vi "Load_Digital_OP.vi"(7 "ReadOnlyIn":T11={"Qref"={"ValveCTR"=refnum, "Error"=refnum}, "UI_EN"=FALSE, "UserEventREF"={"TimeBasedProducer"={"Reg"=refnum, "Ref"=refnum}, "TimeBasedTempRead"={"Reg"=refnum, "Ref"=refnum}}, "UI_REF"=variant(cluster{} {}), "Paths"={"Log_Dir"=path "", "TempLog"=path "", "WateringLog"=path "", "Error"=path "", "Settings_Dir"=path "", "CFG.ini"=path "", "Plant_Digital_OP"=path "", "TimeTable"=path "", "Consol_Dir"=path "", "Input"=path "", "Output"=path "", "Timeout"=path "", "TimeoutTable"=path "", "Ch_Stat"=path "", "Temp"=path ""}, "PI_REF"={"IO"=enum."Remote", "Interface"=enum."Serial", "LINX Device Config"={"Interface"=enum."Serial", "COM Port"="COM13", "TCP Configuration"={"IP Address"="", "Port"=0}, "Device Family"=1, "Device ID"=1, "Device Name"="myRIO-1900", "TCP Ref"=refnum, "Channels"={"DI"=[0, 1, 2, 3, 4, 5, 6, 7, 8, 9, 10, 11, 12, 13, 14, 15, 16, 17, 18, 19, 20, 21, 22, 23, 24, 25, 26, 27, 28, 29, 30, 31, 32, 33, 34, 35, 36, 37, 38, 39, 40, 41, 42, 43, 44, 45, 46], "DO"=[0, 1, 2, 3, 4, 5, 6, 7, 8, 9, 10, 11, 12, 13, 14, 15, 16, 17, 18, 19, 20, 21, 22, 23, 24, 25, 26, 27, 28, 29, 30, 31, 32, 33, 34, 35, 36, 37, 38, 39, 40, 41, 42, 43, 44, 45, 46], "AI"=[0, 1, 2, 3, 4, 5, 6, 7, 8, 9, 10, 11], "AO"=[], "PWM"=[3, 5, 6, 9, 10], "QE"=[], "UART"=[0, 1], "I2C 2"=[0], "SPI"=[0], "CAN"=[], "Servo"=[], "AI Ref (V)"=0.0, "AI Resolution (Bits)"=0, "AO Ref (V)"=0.0, "AO Resolution (Bits)"=0}}}, "CFG"={"ProducerEn_PC"=FALSE, "Producer_PC_ms"=0, "ProducerEn_PI"=FALSE, "Producer_PI_ms"=0, "TempLogInterval"=15, "SystemResetTime"=0.0}} {"CFG"."SystemResetTime" format="%<%H:%M:%S>t"}, 8 "Error In":errorcluster, 9 "Oper":enum16{"FromFile", "FromMem"}(ring), 10 "Plants_Digital_OP":refnum<vi>, 11 "Read_WriteIN":T2={"Time Table"=[{"Set Time"=0.0, "Control"=enum."Time", "Duration[S]"=3.0, "Liter"=0.0, "Plant Name."="", "Watered"=FALSE, "Su"=FALSE, "Mo"=FALSE, "Tu"=FALSE, "We"=FALSE, "Th"=FALSE, "Fr"=FALSE, "Sa"=FALSE}, {"Set Time"=0.0, "Control"=enum."Time", "Duration[S]"=5.0, "Liter"=0.0, "Plant Name."="", "Watered"=FALSE, "Su"=FALSE, "Mo"=FALSE, "Tu"=FALSE, "We"=FALSE, "Th"=FALSE, "Fr"=FALSE, "Sa"=FALSE}, {"Set Time"=0.0, "Control"=enum."Time", "Duration[S]"=5.0, "Liter"=0.0, "Plant Name."="", "Watered"=FALSE, "Su"=FALSE, "Mo"=FALSE, "Tu"=FALSE, "We"=FALSE, "Th"=FALSE, "Fr"=FALSE, "Sa"=FALSE}], "Plants_Digital_OP"=[], "delta_ms_w_Index"={"delta_ms"=[], "Index"=[], "RunArray"=[]}, "TimeOutInfo"={"Timeout"=0, "ValveCTR"={"State"=enum."Open Valve", "Channel No"=0, "Duration[S]"=0.0}, "Index"=0}, "LoopName"=""} {"TimeOutInfo"."ValveCTR"."Channel No" items=["7"=7, "11"=11, "12"=12, "13"=13, "15"=15, "16"=16, "18"=18, "29"=29, "32"=32, "33"=33, "35"=35, "36"=36, "37"=37, "38"=38, "40"=40]; "delta_ms_w_Index"."RunArray"."Channel No" items=["7"=7, "11"=11, "12"=12, "13"=13, "15"=15, "16"=16, "18"=18, "29"=29, "32"=32, "33"=33, "35"=35, "36"=36, "37"=37, "38"=38, "40"=40]; "Plants_Digital_OP"."Channel No" items=["7"=7, "11"=11, "12"=12, "13"=13, "15"=15, "16"=16, "18"=18, "29"=29, "32"=32, "33"=33, "35"=35, "36"=36, "37"=37, "38"=38, "40"=40]; "Time Table"."Liter" min=0.0; "Time Table"."Set Time" format="%<%H:%M:%S>t"; "Time Table"."Duration[S]" min=0.0}) -> (0 "Error Out":errorcluster, 2 "ValidCh":T1[](array[typedef]) items=["7"=7, "11"=11, "12"=12, "13"=13, "15"=15, "16"=16, "18"=18, "29"=29, "32"=32, "33"=33, "35"=35, "36"=36, "37"=37, "38"=38, "40"=40], 3 "Read_WriteIOUT":T2={"Time Table"=[{"Set Time"=0.0, "Control"=enum."Time", "Duration[S]"=3.0, "Liter"=0.0, "Plant Name."="", "Watered"=FALSE, "Su"=FALSE, "Mo"=FALSE, "Tu"=FALSE, "We"=FALSE, "Th"=FALSE, "Fr"=FALSE, "Sa"=FALSE}, {"Set Time"=0.0, "Control"=enum."Time", "Duration[S]"=5.0, "Liter"=0.0, "Plant Name."="", "Watered"=FALSE, "Su"=FALSE, "Mo"=FALSE, "Tu"=FALSE, "We"=FALSE, "Th"=FALSE, "Fr"=FALSE, "Sa"=FALSE}, {"Set Time"=0.0, "Control"=enum."Time", "Duration[S]"=5.0, "Liter"=0.0, "Plant Name."="", "Watered"=FALSE, "Su"=FALSE, "Mo"=FALSE, "Tu"=FALSE, "We"=FALSE, "Th"=FALSE, "Fr"=FALSE, "Sa"=FALSE}], "Plants_Digital_OP"=[], "delta_ms_w_Index"={"delta_ms"=[], "Index"=[], "RunArray"=[]}, "TimeOutInfo"={"Timeout"=0, "ValveCTR"={"State"=enum."Open Valve", "Channel No"=0, "Duration[S]"=0.0}, "Index"=0}, "LoopName"=""} {"TimeOutInfo"."ValveCTR"."Channel No" items=["7"=7, "11"=11, "12"=12, "13"=13, "15"=15, "16"=16, "18"=18, "29"=29, "32"=32, "33"=33, "35"=35, "36"=36, "37"=37, "38"=38, "40"=40]; "delta_ms_w_Index"."RunArray"."Channel No" items=["7"=7, "11"=11, "12"=12, "13"=13, "15"=15, "16"=16, "18"=18, "29"=29, "32"=32, "33"=33, "35"=35, "36"=36, "37"=37, "38"=38, "40"=40]; "Plants_Digital_OP"."Channel No" items=["7"=7, "11"=11, "12"=12, "13"=13, "15"=15, "16"=16, "18"=18, "29"=29, "32"=32, "33"=33, "35"=35, "36"=36, "37"=37, "38"=38, "40"=40]; "Time Table"."Liter" min=0.0; "Time Table"."Set Time" format="%<%H:%M:%S>t"; "Time Table"."Duration[S]" min=0.0})   [LabVIEW 2014, in "TimeBasedProd.lvlib"]
uses:
  TimeBasedProd.lvlib
  TypeDef/Read_Write.ctl
  TimeTable/TypeDef/Time_Table.ctl
  TimeTable/TypeDef/Time_Table_CTR.ctl
  TypeDef/Plant_OP_Map.ctl
  TypeDef/Plant_OP_Map_CTR.ctl
  ValveCTRL/TypeDef/CHs_List.ctl
  TypeDef/TimeOutInfo.ctl
  ValveCTRL/TypeDef/Queue_Cluster.ctl
  ValveCTRL/TypeDef/States_Enum.ctl
  TypeDef/UpdateTimeOutinfo.ctl
  Main/TypeDef/ReadOnly.ctl
  Main/TypeDef/EventData.ctl
  <vilib>/MakerHub/LINX/Private/Type Defs/LINX Ref.ctl
  <vilib>/MakerHub/LINX/Private/Type Defs/Platform.ctl
  <vilib>/MakerHub/LINX/Private/Type Defs/Interface.ctl
  <vilib>/MakerHub/LINX/Private/Device/Type Defs/LINX Device Config.ctl
  <vilib>/MakerHub/LINX/Private/Device/Type Defs/TCP Config.ctl
  <vilib>/MakerHub/LINX/Private/Device/Type Defs/Channels.ctl
  Main/Init/ReadInitCFG/TypeDef/CFG_Cluster.ctl
  ValveCTRL/ValveCTRL.lvlib
  Main/Main.lvlib
  <vilib>/MakerHub/LINX/LMH-LINX.lvlib
  <vilib>/MakerHub/LINX/Private/Device/Device.lvlib
panel:
  # "Watering Days"
  # "Watering Days"
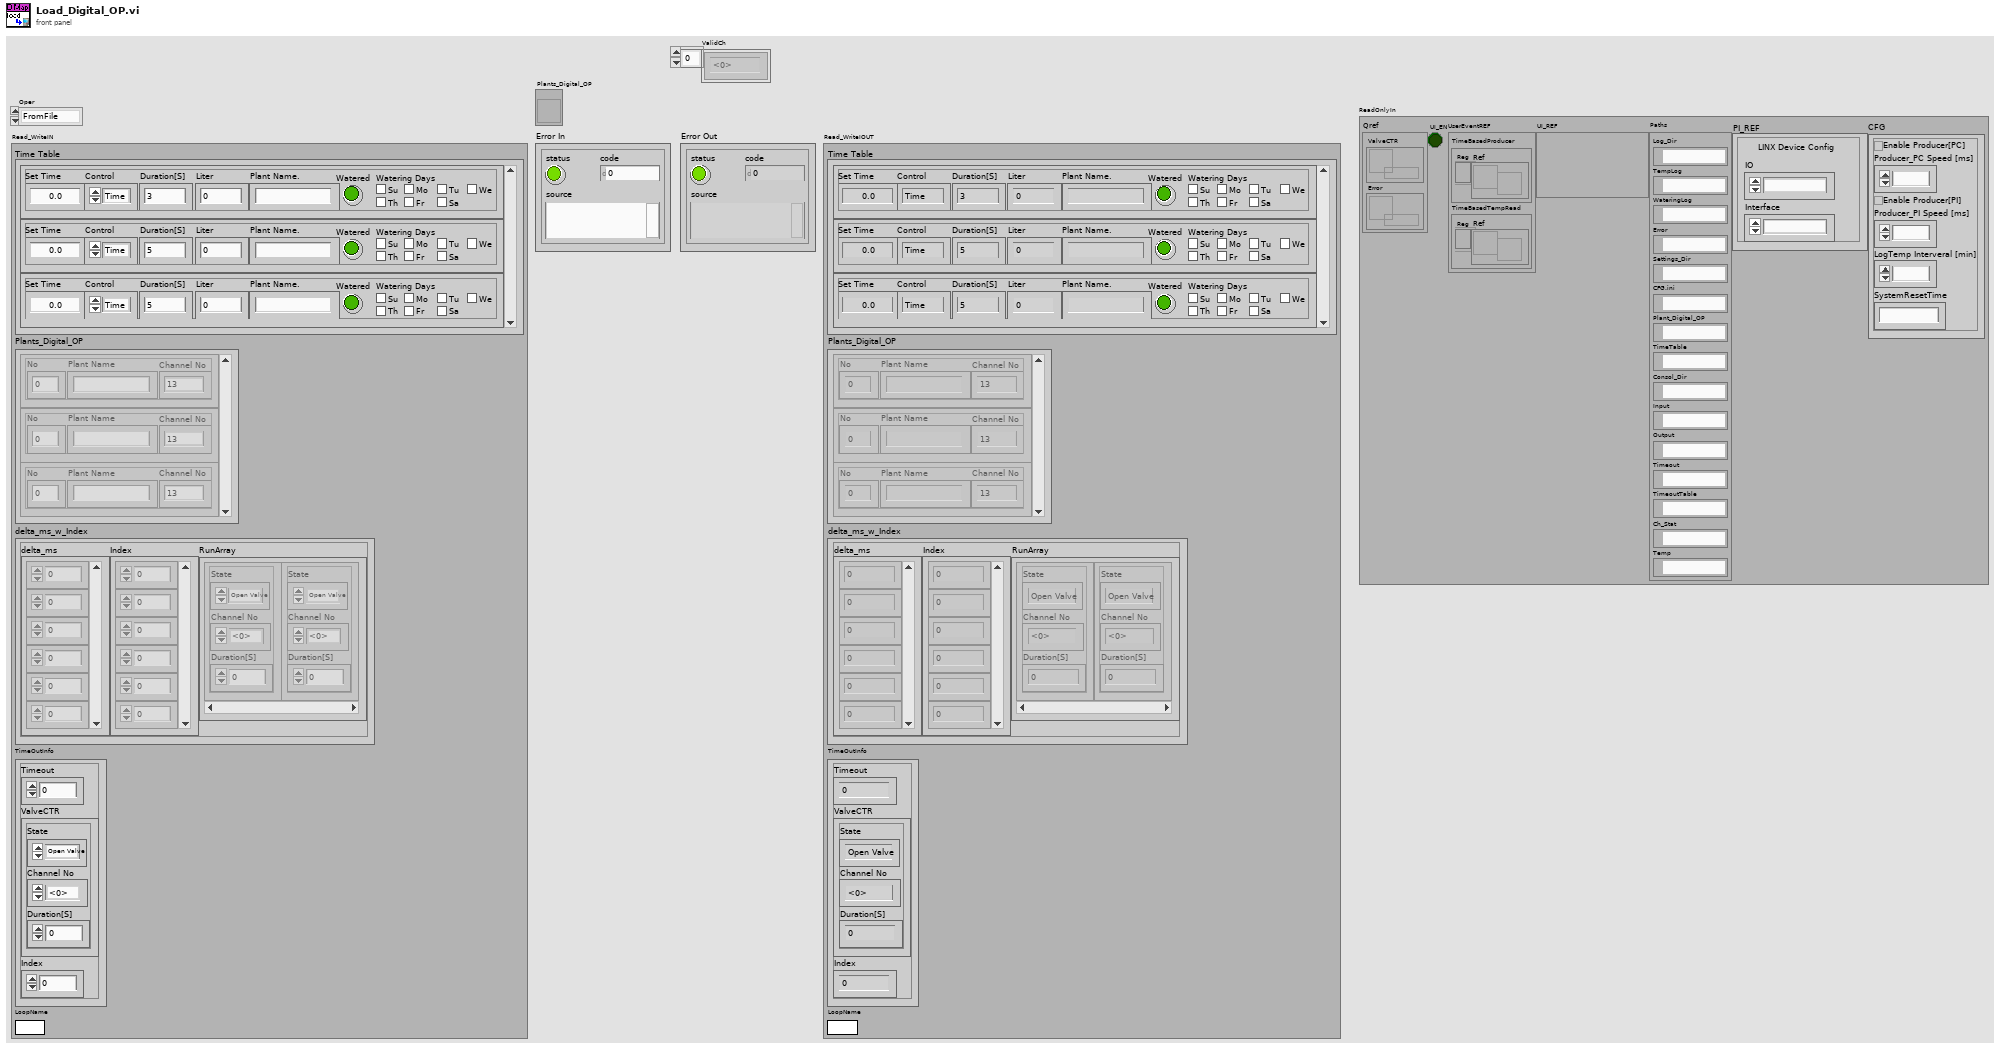
[diagram p1: front panel]
types:
  T1 = typedef "ValveCTRL.lvlib/CHs_List.ctl" = u8
  T2 = typedef "TimeBasedProd.lvlib/Read_Write.ctl" = cluster{"Time Table":T3, "Plants_Digital_OP":T5, "delta_ms_w_Index":T7, "TimeOutInfo":T10, "LoopName":string}
  T3 = typedef "TimeBasedProd.lvlib/Time_Table.ctl" = T4[]
  T4 = typedef "TimeBasedProd.lvlib/Time_Table_CTR.ctl" = cluster{"Set Time":dbl, "Control":enum16{"Time", "Flow"}, "Duration[S]":dbl, "Liter":dbl, "Plant Name.":string, "Watered":bool, "Su":bool, "Mo":bool, "Tu":bool, "We":bool, "Th":bool, "Fr":bool, "Sa":bool}
  T5 = typedef "TimeBasedProd.lvlib/Plant_OP_Map.ctl" = T6[]
  T6 = typedef "TimeBasedProd.lvlib/Plant_OP_Map_CTR.ctl" = cluster{"No":u8, "Plant Name":string, "Channel No":T1}
  T7 = typedef "TimeBasedProd.lvlib/TimeOutInfo.ctl" = cluster{"delta_ms":i32[], "Index":i32[], "RunArray":T8[]}
  T8 = typedef "ValveCTRL.lvlib/Queue_Cluster.ctl" = cluster{"State":T9, "Channel No":T1, "Duration[S]":dbl}
  T9 = typedef "ValveCTRL.lvlib/States_Enum.ctl" = enum16{"Open Pump", "Open Valve", "Wait Valve", "Close Pump", "Close Valve", "Save State", "StopLoop", "ValidCh"}
  T10 = typedef "TimeBasedProd.lvlib/UpdateTimeOutinfo.ctl" = cluster{"Timeout":i32, "ValveCTR":T8, "Index":i32}
  T11 = typedef "Main.lvlib/ReadOnly.ctl" = cluster{"Qref":cluster{"ValveCTR":refnum<queue>, "Error":refnum<queue>}, "UI_EN":bool, "UserEventREF":cluster{"TimeBasedProducer":cluster{"Reg":refnum<event-registration>, "Ref":refnum<user-event>}, "TimeBasedTempRead":cluster{"Reg":refnum<event-registration>, "Ref":refnum<user-event>}}, "UI_REF":variant, "Paths":cluster{"Log_Dir":path, "TempLog":path, "WateringLog":path, "Error":path, "Settings_Dir":path, "CFG.ini":path, "Plant_Digital_OP":path, "TimeTable":path, "Consol_Dir":path, "Input":path, "Output":path, "Timeout":path, "TimeoutTable":path, "Ch_Stat":path, "Temp":path}, "PI_REF":T12, "CFG":T18}
  T12 = typedef "LMH-LINX.lvlib/LINX Ref.ctl" = cluster{"IO":T13, "Interface":T14, "LINX Device Config":T15}
  T13 = typedef "LMH-LINX.lvlib/Platform.ctl" = enum16{"Remote", "Local"}
  T14 = typedef "LMH-LINX.lvlib/Interface.ctl" = enum16{"Serial", "TCP"}
  T15 = typedef "LMH-LINX.lvlib/Device.lvlib/LINX Device Config.ctl" = cluster{"Interface":T14, "COM Port":refnum<visa-resource-name>, "TCP Configuration":T16, "Device Family":u8, "Device ID":u8, "Device Name":string, "TCP Ref":refnum<k5>, "Channels":T17}
  T16 = typedef "LMH-LINX.lvlib/Device.lvlib/TCP Config.ctl" = cluster{"IP Address":string, "Port":u16}
  T17 = typedef "LMH-LINX.lvlib/Channels.ctl" = cluster{"DI":u8[], "DO":u8[], "AI":u8[], "AO":u8[], "PWM":u8[], "QE":u8[], "UART":u8[], "I2C 2":u8[], "SPI":u8[], "CAN":u8[], "Servo":u8[], "AI Ref (V)":dbl, "AI Resolution (Bits)":u8, "AO Ref (V)":dbl, "AO Resolution (Bits)":u8}
  T18 = typedef "Main.lvlib/CFG_Cluster.ctl" = cluster{"ProducerEn_PC":bool, "Producer_PC_ms":u32, "ProducerEn_PI":bool, "Producer_PI_ms":u32, "TempLogInterval":u32, "SystemResetTime":dbl}
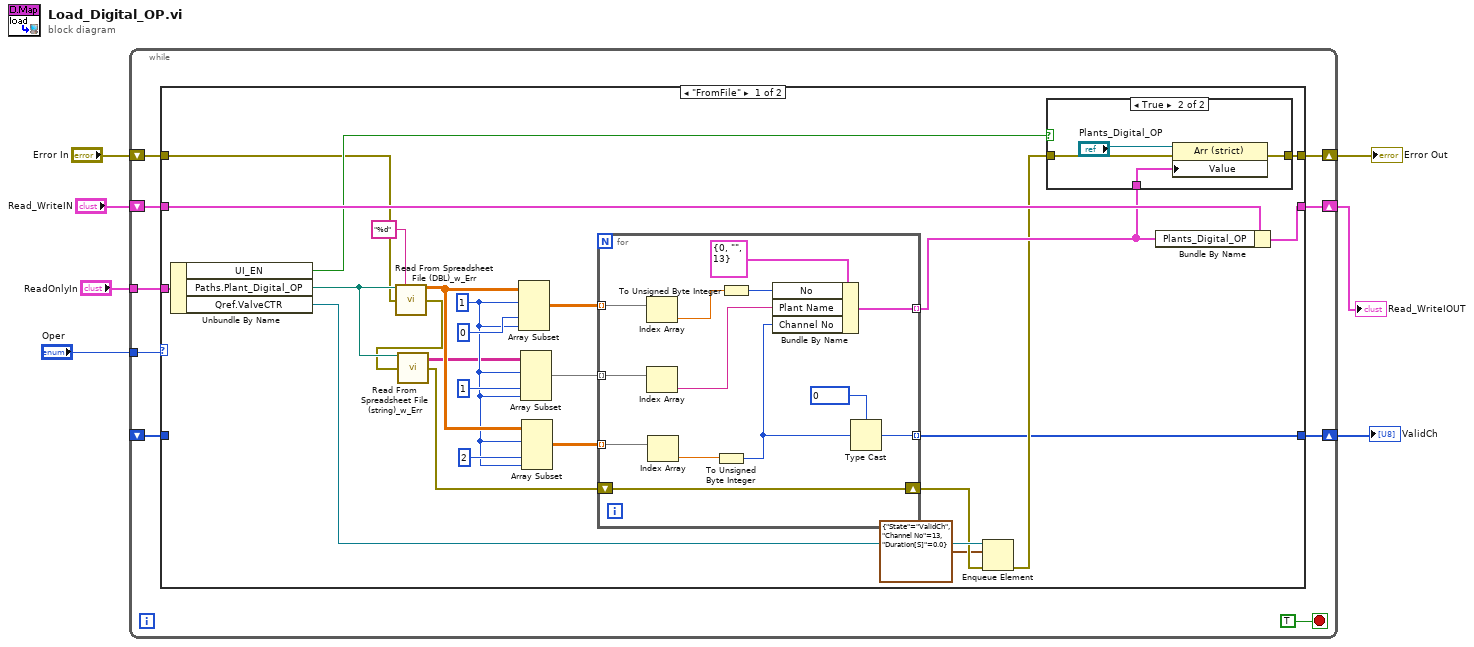
[diagram p0: block diagram]
diagram:
  n1 = while {
    tunnel: "ReadOnlyIn" -> [w16]
    shift-right: [w14] -> w5
    shift-left: "Read_WriteIN" -> [w15]
    shift-right: [w13] -> w4
    shift-left: "Error In" -> [w12]
    shift-right: [w10] -> w2
    shift-left: _ -> [w8]
    tunnel: "Oper" -> [w9]
    stop <- TRUE stop-if-true
    n2 = case shown="\"FromFile\"" w9 {
      tunnel: w16 -> [w31 _]
      tunnel: w15 -> [w29 w61]
      tunnel: [w28 w61] -> w14
      tunnel: [w26 w60] -> w13
      tunnel: w12 -> [w23 w60]
      tunnel: [w18 w62] -> w10
      tunnel: w8 -> [_ w62]
      frame "FromFile" {
        w34 = 1 ("index")
        n3 = Unbundle By Name(w31) -> ("UI_EN"=w25:bool, "Paths.Plant_Digital_OP"=w30:path, "Qref.ValveCTR"=w24:refnum<queue>)
        n4 = call "Read From Spreadsheet File (DBL)_w_Err.vi"("file path (dialog if empty)"=w30, "format (%.3f)"="%d", "error in"=w23) -> ("all rows"=w35:dbl[][], "error out"=w22:errorcluster)  [unwired: 7 in, 4 out]
        n5 = call "Read From Spreadsheet File (string)_w_Err.vi"("file path (dialog if empty)"=w30, "error in"=w22) -> ("all rows"=w33:string[][], "error out"=w21:errorcluster)  [unwired: 8 in, 4 out]
        n6 = Array Subset(array=w35, index (row)=w34, index (col)=0 ("index (row)"), length (col)=w34) -> (w38:dbl[][])  [unwired: 1 in]
        n7 = Array Subset(array=w33, index (row)=w34, index (col)=1 ("index"), length (col)=w34) -> (w37:string[][])  [unwired: 1 in]
        n8 = Array Subset(array=w35, index (row)=w34, index (col)=2 ("index"), length (col)=w34) -> (w32:dbl[][])  [unwired: 1 in]
        n9 = for {
          tunnel: w38 -> [w57] mode=indexing
          tunnel: [w59] -> w27 mode=indexing
          tunnel: w37 -> [w58] mode=indexing
          tunnel: w32 -> [w52] mode=indexing
          tunnel: [w48] -> w18 mode=indexing
          shift-right: [w47] -> w20
          shift-left: w21 -> [w47]
          w50 = T1 0 items=["7"=7, "11"=11, "12"=12, "13"=13, "15"=15, "16"=16, "18"=18, "29"=29, "32"=32, "33"=33, "35"=35, "36"=36, "37"=37, "38"=38, "40"=40] ("Channel No")
          n10 = Index Array(array=w57) -> (element=w55:dbl)  [unwired: 1 in]
          n11 = Index Array(array=w58) -> (element=w53:string)  [unwired: 1 in]
          n12 = Index Array(array=w52) -> (element=w51:dbl)  [unwired: 1 in]
          n13 = To Unsigned Byte Integer(number=w51) -> (unsigned 8bit integer=w49:u8)
          n14 = To Unsigned Byte Integer(number=w55) -> (unsigned 8bit integer=w54:u8)
          n15 = Bundle By Name(cluster=T6 {"No"=0, "Plant Name"="", "Channel No"=13} ("Cluster"), "No"=w54, "Plant Name"=w53, "Channel No"=w49) -> (w59:T6)
          n16 = Type Cast(type=w50, x=w49) -> (*(type *) &x=w48:T1)
        }
        n17 = Enqueue Element(queue=w24, element=T8 {"State"=enum."ValidCh", "Channel No"=13, "Duration[S]"=0.0}, error in (no error)=w20) -> (error out=w19:errorcluster)  [unwired: 1 in, 2 out]
        n18 = case shown="True" w25 {
          tunnel: w27 -> [_ w45]
          tunnel: w19 -> [w42 w44]
          tunnel: [w42 w43] -> w26
          frame False {
          }
          frame True {
            n19 = property class="Arr (strict)"(reference="Plants_Digital_OP", error in=w44, "Value"=w45) -> (error out=w43:errorcluster)  [unwired: 1 out]
          }
        }
        n20 = Bundle By Name(cluster=w29, "Plants_Digital_OP"=w27) -> (w28:T2)
      }
      frame "FromMem" {
      }
    }
  }
  "Error Out" <- w4
  "Read_WriteIOUT" <- w5
  "ValidCh" <- w2
